vi "Game Manager.vi"(8 "error in (no error)":errorcluster) -> (0 "error out":errorcluster)   [LabVIEW 2014]
uses:
  Recipe step.ctl
  STD - Tap Mode.ctl
  Globals.vi
panel:
  in  "Recipe queue":refnum<queue>
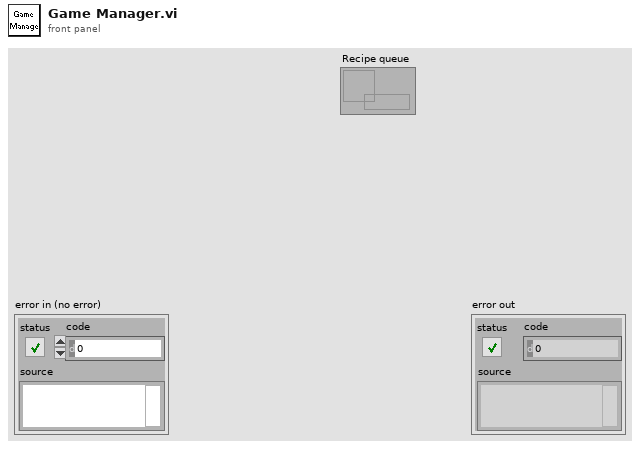
[diagram p1: front panel]
types:
  T1 = typedef "Recipe step.ctl" = cluster{"Control Mode":T2, "Length (s)":dbl}
  T2 = typedef "STD - Tap Mode.ctl" = enum32{"No Action", "Stay Level", "Rise", "Fall", "Calibrate"}
  T3 = typedef "FlappyHeightPoint.ctl" = cluster{"Time (s)":dbl, "Height (px)":dbl}
  T4 = typedef "IMAQ Image.ctl" = refnum<image>
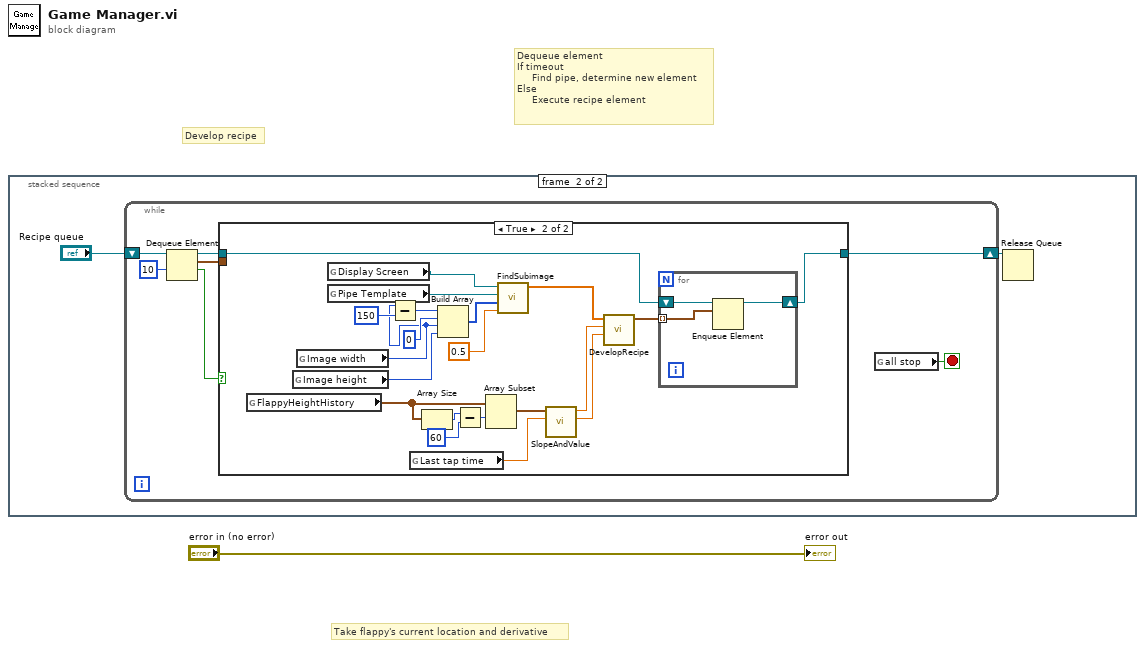
[diagram p0: block diagram]
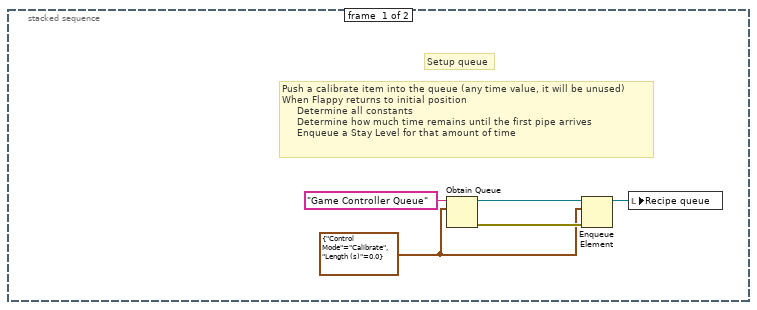
[diagram p2: hidden frame]
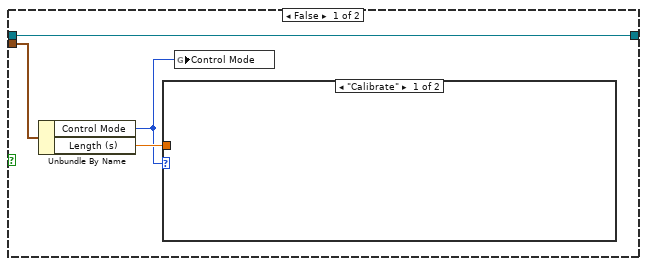
[diagram p3: hidden frame]
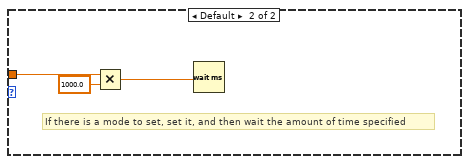
[diagram p4: hidden frame]
diagram:
  # "Develop recipe"
  # "Take flappy's current location and derivative"
  # "Dequeue element\nIf timeout\n     Find pipe, determine new element\nElse\n     Execute recipe element"
  n1 = stacked-sequence {
    frame #0 {
      w3 = T1 {"Control Mode"=enum."Calibrate", "Length (s)"=0.0}
      # "Push a calibrate item into the queue (any time value, it will be unused)\nWhen Flappy returns to initial position\n     Determine all constants\n     Determine how much time remains until the first pipe arrives\n     Enqueue a Stay Level for that amount of time"
      # "Setup queue"
      n2 = Obtain Queue(name (unnamed)="Game Controller Queue", element data type=w3) -> (queue out=w5:refnum<queue>, error out=w4:errorcluster)  [unwired: 3 in, 1 out]
      n3 = Enqueue Element(queue=w5, element=w3, error in (no error)=w4) -> (queue out=w2:refnum<queue>)  [unwired: 1 in, 2 out]
      n4 = local write "Recipe queue"(w2) -> ()
    }
    frame #1 {
      n5 = while {
        shift-right: [w9] -> w7
        shift-left: "Recipe queue" -> [w14]
        stop <- w15 stop-if-true
        n6 = Dequeue Element(queue=w14, timeout in ms (-1)=10) -> (queue out=w10:refnum<queue>, element=w11:T1, timed out?=w12:bool)  [unwired: 1 in, 1 out]
        n7 = case shown="True" w12 {
          tunnel: w11 -> [w19 _]
          tunnel: w10 -> [w17 w28]
          tunnel: [w17 w27] -> w9
          frame False {
            n8 = Unbundle By Name(w19) -> ("Control Mode"=w16:T2, "Length (s)"=w18:dbl)
            n9 = case shown="\"Calibrate\"" w16 {
              tunnel: w18 -> [_ w22]
              frame "Calibrate" {
              }
              frame Default {
                # "If there is a mode to set, set it, and then wait the amount of time specified"
                n10 = Multiply(x=w22, y=1000.0) -> (x*y=w20:dbl)
                n11 = Wait (ms)(milliseconds to wait=w20) -> ()  [unwired: 1 out]
              }
            }
            n12 = global write "Globals.vi" "Control Mode"(w16) -> ()
          }
          frame True {
            n13 = global read "Globals.vi" "FlappyHeightHistory"() -> (w29:T3[])
            n14 = global read "Globals.vi" "Image height"() -> (w33:u32)
            n15 = global read "Globals.vi" "Image width"() -> (w34:u32)
            n16 = global read "Globals.vi" "Display Screen"() -> (w30:T4)
            n17 = global read "Globals.vi" "Pipe Template"() -> (w32:T4)
            n18 = Subtract(x=w34, y=150) -> (x-y=w38:u32)
            n19 = global read "Globals.vi" "Last tap time"() -> (w31:dbl)
            n20 = Array Size(array=w29) -> (size(s)=w43:i32)
            n21 = Build Array(w38, 0 ("element"), w34, w33) -> (w36:u32[])
            n22 = Subtract(x=w43, y=60) -> (x-y=w42:i32)
            n23 = Array Subset(array=w29, index=w42) -> (w40:T3[])  [unwired: 1 in]
            n24 = call "FindSubimage.vi"("Scale factor (1)"=0.5, "ROI (left top right bottom)"=w36, "RGB Template"=w32, "RGB Image"=w30) -> ("Locations (left, top)"=w26:dbl[])  [unwired: 7 in]
            n25 = call "SlopeAndValue.vi"("Threshold time"=w31, "Values History"=w40) -> ("Derivative"=w24:dbl, "Value"=w25:dbl)  [unwired: 8 in]
            n26 = call "DevelopRecipe.vi"("Flappy Velocity"=w24, "Flappy Height"=w25, "Pipe location (left, top)"=w26) -> ("Recipe"=w23:T1[])  [unwired: 8 in]
            n27 = for {
              shift-right: [w45] -> w27
              shift-left: w28 -> [w46]
              tunnel: w23 -> [w44] mode=indexing
              n28 = Enqueue Element(queue=w46, element=w44) -> (queue out=w45:refnum<queue>)  [unwired: 2 in, 2 out]
            }
          }
        }
        n29 = global read "Globals.vi" "all stop"() -> (w15:bool)
      }
      n30 = Release Queue(queue=w7) -> ()  [unwired: 2 in, 3 out]
    }
  }
  "error out" <- "error in (no error)"
